vi "Servo(putinloop).vi"(8 "Count(uSec)":u16=1500, 11 "FPGA I/O Out":refnum<k21>="Port0/DIO0") -> ()   [LabVIEW 2011, in "kevLib2011.lvlib"]
uses:
  kevLib2011.lvlib
  <vilib>/eio/EIONode/EIONode.xnode
  <vilib>/rvi/eio/common/nirviEmuTemplateMethod_errors.vi
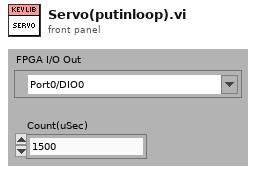
[diagram p1: front panel]
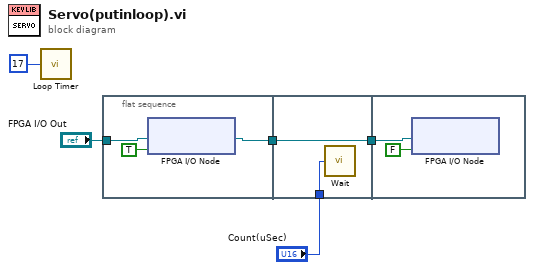
[diagram p0: block diagram]
diagram:
  n1 = call "Loop Timer"("Count(mSec)"=u8 17) -> ()  [unwired: 1 out]
  n2 = flat-sequence {
    tunnel: [w7] -> w5
    tunnel: "FPGA I/O Out" -> [w8]
    tunnel: w5 -> [w10]
    tunnel: [w10] -> w4
    tunnel: "Count(uSec)" -> [w9]
    tunnel: w4 -> [w12]
    frame #0 {
      n3 = xnode "FPGA I/O Node"("I/O Item"=TRUE, "FPGA I/O In"=w8) -> ("FPGA I/O Out"=w7:refnum<k21>)
    }
    frame #1 {
      n4 = call "Wait"("Count(uSec)"=w9) -> ()  [unwired: 1 out]
    }
    frame #2 {
      n5 = xnode "FPGA I/O Node"("I/O Item"=FALSE, "FPGA I/O In"=w12) -> ()  [unwired: 1 out]
    }
  }
